vi "MGCC_Control.vi"() -> ()   [LabVIEW 2016]
panel:
  out "LC_Vol":dbl
  out "LC_Status":dbl
  out "LC_Re_Pwr":dbl
  out "LC_Pwr":dbl
  out "LC_Freq":dbl
  out "LC_Error":dbl
  out "LC_BESS_SOC":dbl
  in  "LC_Pwr_Ref":dbl
  in  "LC_Error_Clear":bool
  in  "LC_Vol_Ref":dbl
  in  "LC_Sync_Mag_Diff":dbl
  in  "LC_Sync_Freq_Diff":dbl
  in  "LC_Sync_Ang_Diff":dbl
  in  "LC_Status_Cmd":dbl
  in  "LC_Re_Pwr_Ref":dbl
  in  "LC_Freq_Ref":dbl
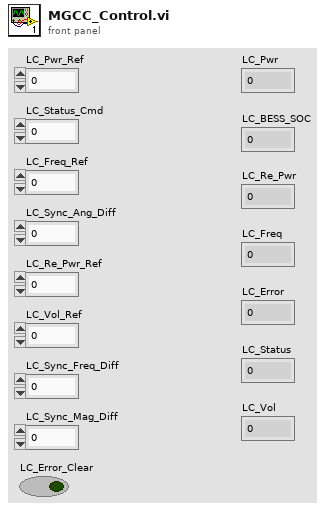
[diagram p1: front panel]
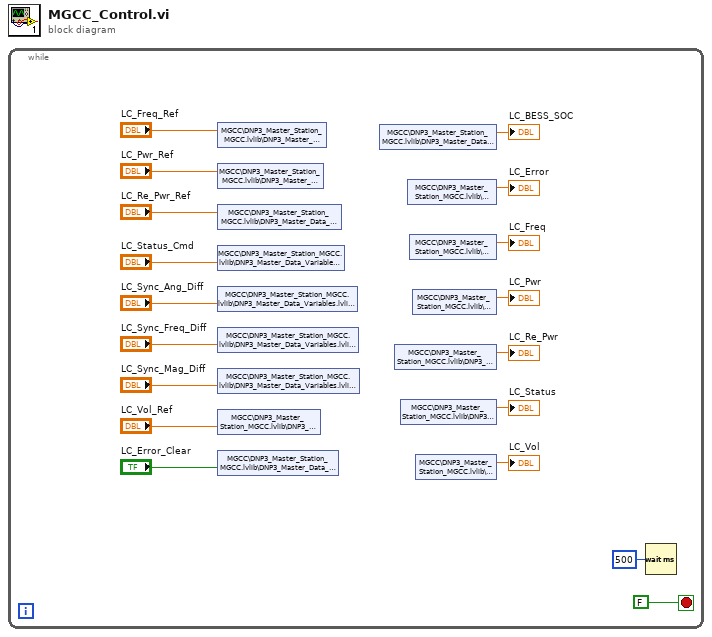
[diagram p0: block diagram]
diagram:
  n1 = while {
    stop <- FALSE stop-if-true
    n2 = shared-variable "MGCC\\DNP3_Master_Station_MGCC.lvlib\\DNP3_Master_Data_Variables.lvlib\\MS_Analog_Control.lvlib\\LC_Freq_Ref"("LC_Freq_Ref") -> ()  [unwired: 1 in, 1 out]
    n3 = shared-variable "MGCC\\DNP3_Master_Station_MGCC.lvlib\\DNP3_Master_Data_Variables.lvlib\\MS_Analog_Control.lvlib\\LC_Pwr_Ref"("LC_Pwr_Ref") -> ()  [unwired: 1 in, 1 out]
    n4 = shared-variable "MGCC\\DNP3_Master_Station_MGCC.lvlib\\DNP3_Master_Data_Variables.lvlib\\MS_Analog_Control.lvlib\\LC_Re_Pwr_Ref"("LC_Re_Pwr_Ref") -> ()  [unwired: 1 in, 1 out]
    n5 = shared-variable "MGCC\\DNP3_Master_Station_MGCC.lvlib\\DNP3_Master_Data_Variables.lvlib\\MS_Analog_Control.lvlib\\LC_Status_Cmd"("LC_Status_Cmd") -> ()  [unwired: 1 in, 1 out]
    n6 = shared-variable "MGCC\\DNP3_Master_Station_MGCC.lvlib\\DNP3_Master_Data_Variables.lvlib\\MS_Analog_Control.lvlib\\LC_Sync_Ang_Diff"("LC_Sync_Ang_Diff") -> ()  [unwired: 1 in, 1 out]
    n7 = shared-variable "MGCC\\DNP3_Master_Station_MGCC.lvlib\\DNP3_Master_Data_Variables.lvlib\\MS_Analog_Control.lvlib\\LC_Sync_Freq_Diff"("LC_Sync_Freq_Diff") -> ()  [unwired: 1 in, 1 out]
    n8 = shared-variable "MGCC\\DNP3_Master_Station_MGCC.lvlib\\DNP3_Master_Data_Variables.lvlib\\MS_Analog_Control.lvlib\\LC_Sync_Mag_Diff"("LC_Sync_Mag_Diff") -> ()  [unwired: 1 in, 1 out]
    n9 = shared-variable "MGCC\\DNP3_Master_Station_MGCC.lvlib\\DNP3_Master_Data_Variables.lvlib\\MS_Analog_Control.lvlib\\LC_Vol_Ref"("LC_Vol_Ref") -> ()  [unwired: 1 in, 1 out]
    n10 = shared-variable "MGCC\\DNP3_Master_Station_MGCC.lvlib\\DNP3_Master_Data_Variables.lvlib\\MS_Binary_Control.lvlib\\LC_Error_Clear"("LC_Error_Clear") -> ()  [unwired: 1 in, 1 out]
    n11 = shared-variable "MGCC\\DNP3_Master_Station_MGCC.lvlib\\DNP3_Master_Data_Variables.lvlib\\MS_Analog_Status.lvlib\\LC_BESS_SOC"() -> (→"LC_BESS_SOC":dbl)  [unwired: 1 in, 1 out]
    n12 = shared-variable "MGCC\\DNP3_Master_Station_MGCC.lvlib\\DNP3_Master_Data_Variables.lvlib\\MS_Analog_Status.lvlib\\LC_Re_Pwr"() -> (→"LC_Re_Pwr":dbl)  [unwired: 1 in, 1 out]
    n13 = shared-variable "MGCC\\DNP3_Master_Station_MGCC.lvlib\\DNP3_Master_Data_Variables.lvlib\\MS_Analog_Status.lvlib\\LC_Status"() -> (→"LC_Status":dbl)  [unwired: 1 in, 1 out]
    n14 = shared-variable "MGCC\\DNP3_Master_Station_MGCC.lvlib\\DNP3_Master_Data_Variables.lvlib\\MS_Analog_Status.lvlib\\LC_Error"() -> (→"LC_Error":dbl)  [unwired: 1 in, 1 out]
    n15 = shared-variable "MGCC\\DNP3_Master_Station_MGCC.lvlib\\DNP3_Master_Data_Variables.lvlib\\MS_Analog_Status.lvlib\\LC_Freq"() -> (→"LC_Freq":dbl)  [unwired: 1 in, 1 out]
    n16 = shared-variable "MGCC\\DNP3_Master_Station_MGCC.lvlib\\DNP3_Master_Data_Variables.lvlib\\MS_Analog_Status.lvlib\\LC_Pwr"() -> (→"LC_Pwr":dbl)  [unwired: 1 in, 1 out]
    n17 = shared-variable "MGCC\\DNP3_Master_Station_MGCC.lvlib\\DNP3_Master_Data_Variables.lvlib\\MS_Analog_Status.lvlib\\LC_Vol"() -> (→"LC_Vol":dbl)  [unwired: 1 in, 1 out]
    n18 = Wait (ms)(milliseconds to wait=u32 500) -> ()  [unwired: 1 out]
  }
